vi "project 3.vi"() -> ()   [LabVIEW 2014]
panel:
  out "correct":i32
  in  "stop game":bool
  out "status":string
  out "numLights":i32
  out "Index":i32
  in  "Green input":bool
  out "user generate":dbl[](array[numeric])
  in  "White input":bool
  in  "Blue input":bool
  in  "Red Input":bool
  out "computer generate":dbl[](array[numeric])
  out "White LED":bool
  out "Blue LED":bool
  out "Red LED":bool
  out "Green LED":bool
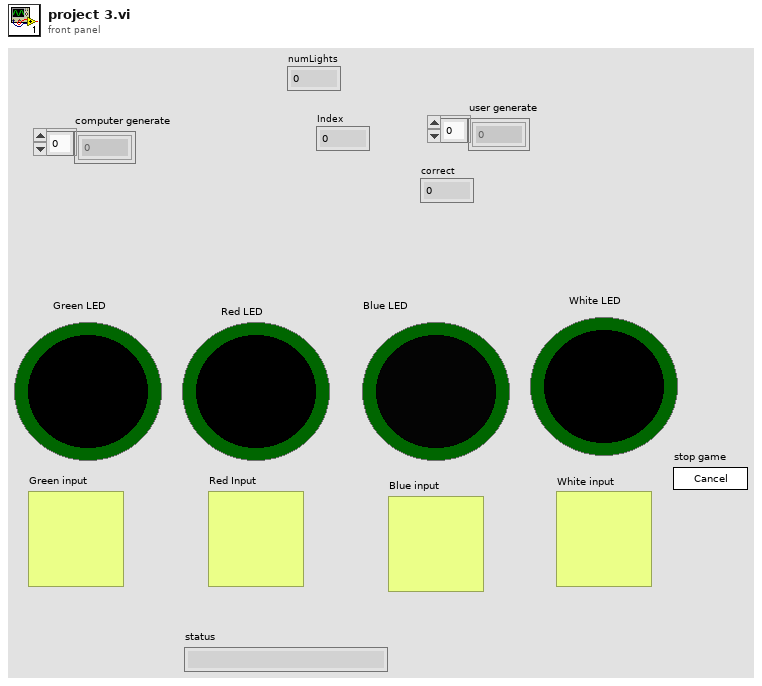
[diagram p1: front panel]
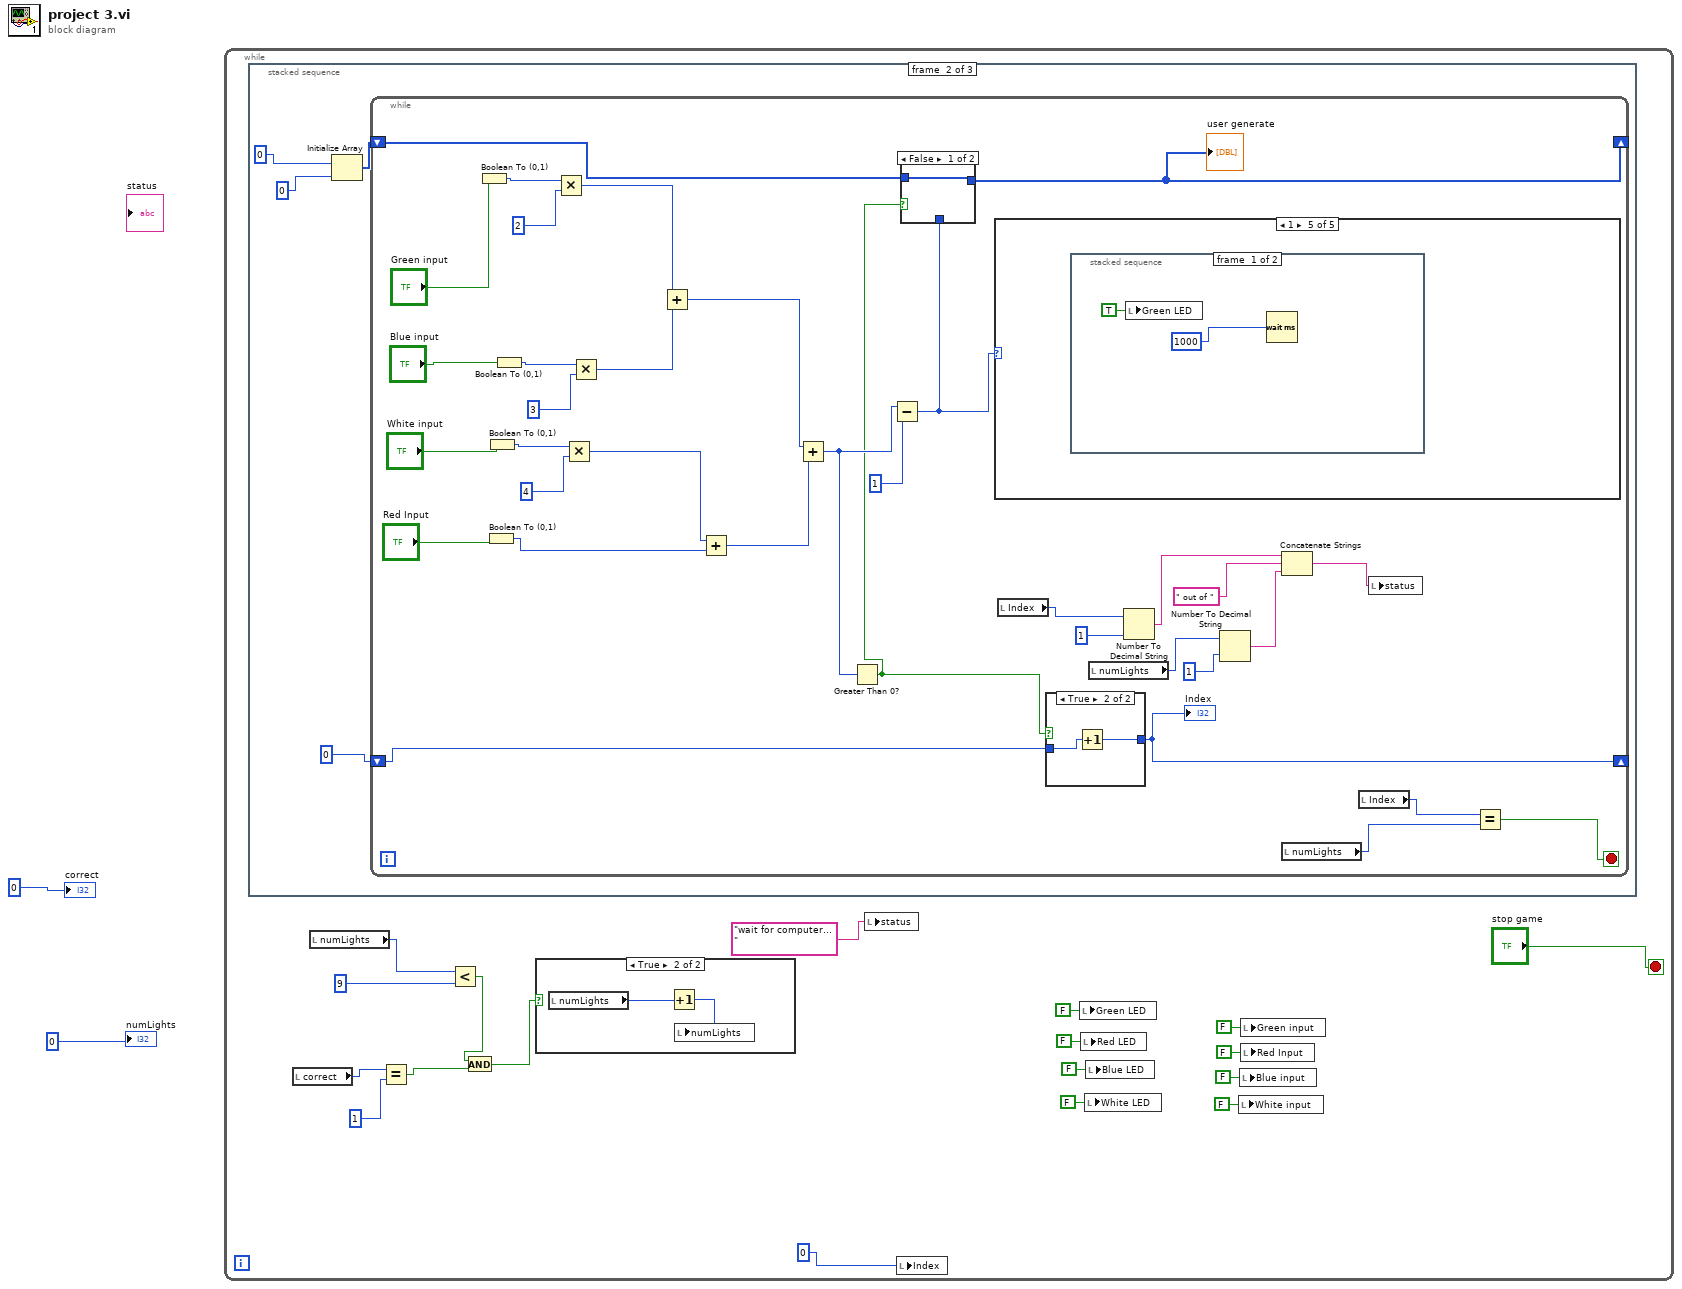
[diagram p0: block diagram]
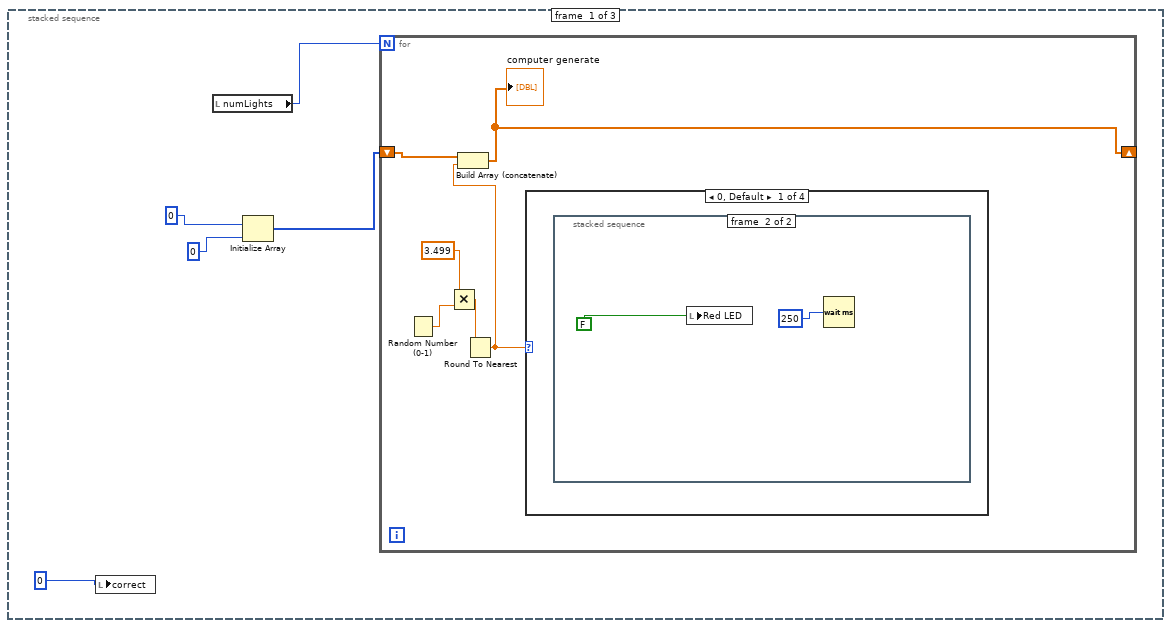
[diagram p3: hidden frame]
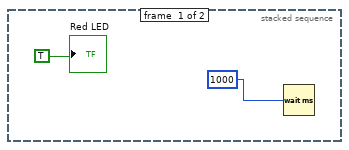
[diagram p4: hidden frame]
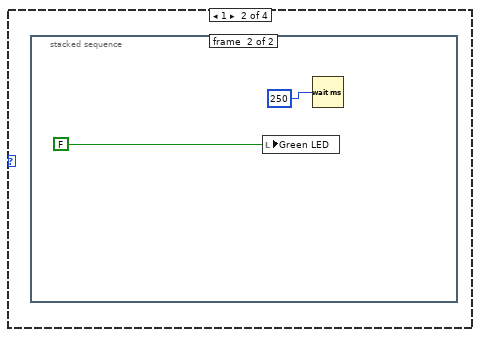
[diagram p5: hidden frame]
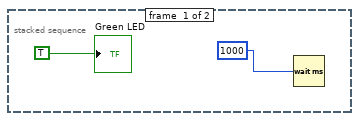
[diagram p6: hidden frame]
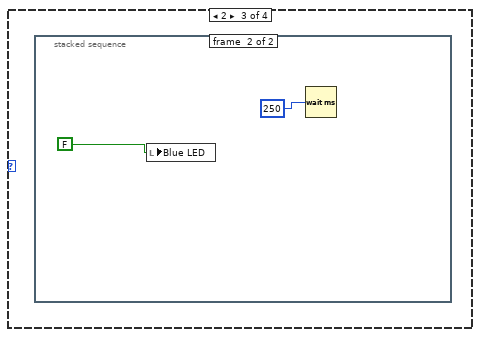
[diagram p7: hidden frame]
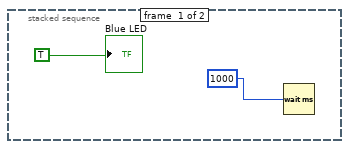
[diagram p8: hidden frame]
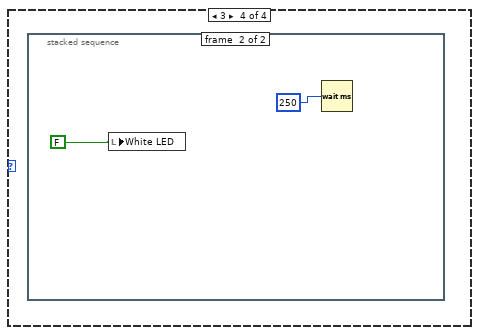
[diagram p9: hidden frame]
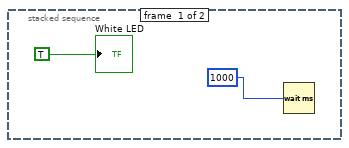
[diagram p10: hidden frame]
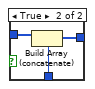
[diagram p11: hidden frame]
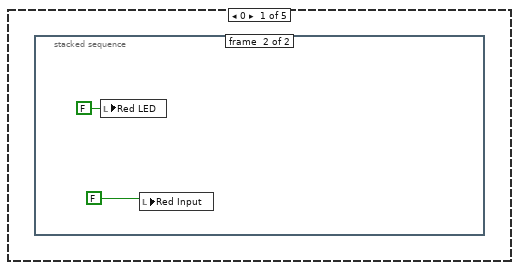
[diagram p13: hidden frame]
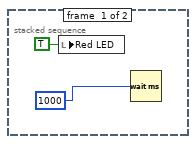
[diagram p14: hidden frame]
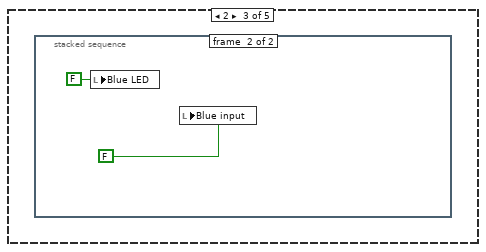
[diagram p16: hidden frame]
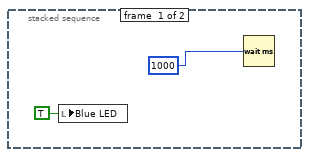
[diagram p17: hidden frame]
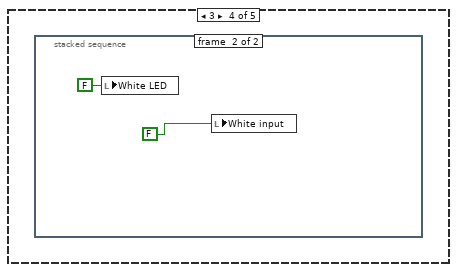
[diagram p18: hidden frame]
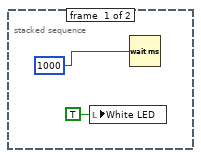
[diagram p19: hidden frame]
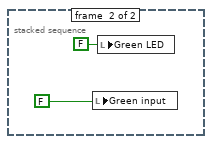
[diagram p20: hidden frame]
diagram:
  n1 = while {
    stop <- "stop game" stop-if-true
    n2 = stacked-sequence {
      frame #0 {
        n3 = local write "correct"(0) -> ()
        n4 = local read "numLights"() -> (w24:i32)
        n5 = Initialize Array(0, 0) -> (w25:i32[])
        n6 = for {
          N: w24 -> [_]
          shift-right: [w28] -> _
          shift-left: w25 -> [w29]
          n7 = Random Number (0-1)() -> (number: 0 to 1=w33:dbl)
          n8 = Multiply(x=3.499, y=w33) -> (x*y=w31:dbl)
          n9 = Round To Nearest(number=w31) -> (nearest integer value=w30:dbl)
          n10 = Build Array (concatenate)(w29, w30) -> (w28:dbl[])
          "computer generate" <- w28
          n11 = case shown="0, Default" w30 {
            frame 0, Default {
              n12 = stacked-sequence {
                frame #0 {
                  n13 = Wait (ms)(milliseconds to wait=1000) -> ()  [unwired: 1 out]
                  "Red LED" <- TRUE
                }
                frame #1 {
                  n14 = local write "Red LED"(FALSE) -> ()
                  n15 = Wait (ms)(milliseconds to wait=250) -> ()  [unwired: 1 out]
                }
              }
            }
            frame 1 {
              n16 = stacked-sequence {
                frame #0 {
                  n17 = Wait (ms)(milliseconds to wait=1000) -> ()  [unwired: 1 out]
                  "Green LED" <- TRUE
                }
                frame #1 {
                  n18 = local write "Green LED"(FALSE) -> ()
                  n19 = Wait (ms)(milliseconds to wait=250) -> ()  [unwired: 1 out]
                }
              }
            }
            frame 2 {
              n20 = stacked-sequence {
                frame #0 {
                  n21 = Wait (ms)(milliseconds to wait=1000) -> ()  [unwired: 1 out]
                  "Blue LED" <- TRUE
                }
                frame #1 {
                  n22 = local write "Blue LED"(FALSE) -> ()
                  n23 = Wait (ms)(milliseconds to wait=250) -> ()  [unwired: 1 out]
                }
              }
            }
            frame 3 {
              n24 = stacked-sequence {
                frame #0 {
                  n25 = Wait (ms)(milliseconds to wait=1000) -> ()  [unwired: 1 out]
                  "White LED" <- TRUE
                }
                frame #1 {
                  n26 = local write "White LED"(FALSE) -> ()
                  n27 = Wait (ms)(milliseconds to wait=250) -> ()  [unwired: 1 out]
                }
              }
            }
          }
        }
      }
      frame #1 {
        n28 = Initialize Array(0, 0) -> (w50:i32[])
        n29 = while {
          shift-right: [w70] -> _
          shift-left: 0 -> [w71]
          shift-right: [w67] -> _
          shift-left: w50 -> [w68]
          stop <- w60 stop-if-true
          n30 = Boolean To (0,1)(Boolean="Green input") -> (0, 1=w75:i16)
          n31 = Boolean To (0,1)(Boolean="Red Input") -> (0, 1=w63:i16)
          n32 = Boolean To (0,1)(Boolean="White input") -> (0, 1=w82:i16)
          n33 = Boolean To (0,1)(Boolean="Blue input") -> (0, 1=w77:i16)
          n34 = Multiply(x=w75, y=2) -> (x*y=w79:i32)
          n35 = Multiply(x=w82, y=4) -> (x*y=w84:i32)
          n36 = Multiply(x=w77, y=3) -> (x*y=w80:i32)
          n37 = Add(x=w79, y=w80) -> (x+y=w85:i32)
          n38 = Add(x=w84, y=w63) -> (x+y=w86:i32)
          n39 = Add(x=w85, y=w86) -> (x+y=w88:i32)
          n40 = Greater Than 0?(x=w88) -> (x > 0?=w66:bool)
          n41 = Subtract(x=w88, y=1) -> (x-y=w69:i32)
          n42 = case shown="False" w66 {
            tunnel: w69 -> [_ w92]
            tunnel: w68 -> [w89 w91]
            tunnel: [w89 w90] -> w67
            frame False {
            }
            frame True {
              n43 = Build Array (concatenate)(w91, w92) -> (w90:i32[])
            }
          }
          "user generate" <- w67
          n44 = case shown="1" w69 {
            frame 0 {
              n45 = stacked-sequence {
                frame #0 {
                  n46 = local write "Red LED"(TRUE ("Red LED")) -> ()
                  n47 = Wait (ms)(milliseconds to wait=1000) -> ()  [unwired: 1 out]
                }
                frame #1 {
                  n48 = local write "Red LED"(FALSE ("Red LED")) -> ()
                  n49 = local write "Red Input"(FALSE) -> ()
                }
              }
            }
            frame Default {
            }
            frame 2 {
              n50 = stacked-sequence {
                frame #0 {
                  n51 = local write "Blue LED"(TRUE ("Blue LED")) -> ()
                  n52 = Wait (ms)(milliseconds to wait=1000) -> ()  [unwired: 1 out]
                }
                frame #1 {
                  n53 = local write "Blue LED"(FALSE ("Blue LED")) -> ()
                  n54 = local write "Blue input"(FALSE) -> ()
                }
              }
            }
            frame 3 {
              n55 = stacked-sequence {
                frame #0 {
                  n56 = local write "White LED"(TRUE ("White LED")) -> ()
                  n57 = Wait (ms)(milliseconds to wait=1000) -> ()  [unwired: 1 out]
                }
                frame #1 {
                  n58 = local write "White LED"(FALSE ("White LED")) -> ()
                  n59 = local write "White input"(FALSE) -> ()
                }
              }
            }
            frame 1 {
              n60 = stacked-sequence {
                frame #0 {
                  n61 = local write "Green LED"(TRUE ("Green LED")) -> ()
                  n62 = Wait (ms)(milliseconds to wait=1000) -> ()  [unwired: 1 out]
                }
                frame #1 {
                  n63 = local write "Green input"(FALSE) -> ()
                  n64 = local write "Green LED"(FALSE ("Green LED")) -> ()
                }
              }
            }
          }
          n65 = local read "Index"() -> (w64:i32)
          n66 = case shown="True" w66 {
            tunnel: [w93 w95] -> w70
            tunnel: w71 -> [w93 w94]
            frame False {
            }
            frame True {
              n67 = Increment(x=w94) -> (x+1=w95:i32)
            }
          }
          "Index" <- w70
          n68 = local read "numLights"() -> (w56:i32)
          n69 = Number To Decimal String(number=w64, width (-)=1) -> (decimal integer string=w59:string)
          n70 = Number To Decimal String(number=w56, width (-)=1) -> (decimal integer string=w54:string)
          n71 = Concatenate Strings(w59, " out of ", w54) -> (w57:string)
          n72 = local read "numLights"() -> (w61:i32)
          n73 = local read "Index"() -> (w62:i32)
          n74 = local write "status"(w57) -> ()
          n75 = Equal?(x=w62, y=w61) -> (x = y?=w60:bool)
        }
      }
      frame #2 {
        n76 = local read "numLights"() -> (w117:i32)
        n77 = local read "user generate"() -> (w118:dbl[])
        n78 = local read "computer generate"() -> (w120:dbl[])
        n79 = local read "numLights"() -> (w121:i32)
        n80 = Array Subset(array=w118, index=0, length=w117) -> (w115:dbl[])
        n81 = Array Subset(array=w120, index=0, length=w121) -> (w116:dbl[])
        n82 = Equal?(x=w116, y=w115) -> (x = y?=w114:bool[])
        n83 = And Array Elements(Boolean array=w114) -> (logical AND=w113:bool)
        n84 = Wait (ms)(milliseconds to wait=2000) -> ()  [unwired: 1 out]
        n85 = case shown="False" w113 {
          frame False {
            n86 = local write "correct"(0 ("correct")) -> ()
            n87 = local write "status"("NOPE") -> ()
          }
          frame True {
            n88 = local write "correct"(1 ("correct")) -> ()
            n89 = local write "status"("WOOOOO you did it!") -> ()
          }
        }
      }
    }
    n90 = local read "correct"() -> (w6:i32)
    n91 = local read "numLights"() -> (w18:i32)
    n92 = Equal?(x=w6, y=1) -> (x = y?=w4:bool)
    n93 = Less?(x=w18, y=9) -> (x < y?=w7:bool)
    n94 = And(x=w7, y=w4) -> (x .and. y?=w3:bool)
    n95 = case shown="True" w3 {
      frame False {
      }
      frame True {
        n96 = local read "numLights"() -> (w22:i32)
        n97 = Increment(x=w22) -> (x+1=w21:i32)
        n98 = local write "numLights"(w21) -> ()
      }
    }
    n99 = local write "status"("wait for computer...") -> ()
    n100 = local write "Index"(0) -> ()
    n101 = local write "Green LED"(FALSE ("Green LED")) -> ()
    n102 = local write "Red LED"(FALSE ("Red LED")) -> ()
    n103 = local write "White LED"(FALSE ("White LED")) -> ()
    n104 = local write "Blue LED"(FALSE ("Blue LED")) -> ()
    n105 = local write "White input"(FALSE ("White input")) -> ()
    n106 = local write "Blue input"(FALSE ("Blue input")) -> ()
    n107 = local write "Green input"(FALSE ("Green input")) -> ()
    n108 = local write "Red Input"(FALSE ("Red Input")) -> ()
  }
  "numLights" <- 0
  "correct" <- 0
